vi "运维调试_CODMn.vi"() -> ()   [LabVIEW 2016, in "一代CodMn.lvlib"]
uses:
  <vilib>/Utility/miscctls.llb/LVPointTypeDef.ctl
panel:
  out "W7.13 加热超时":bool
  out "版本号":u32
  in  "滴定曲线界面返回":bool
  in  "滴定曲线":bool
  out "ORP滴定曲线":u16[](graph)
  out "滴定值":sgl
  out "硫酸计数":u16
  out "草酸钠计数":u16
  out "高锰酸钾计数":u16
  out "进样计数":u16
  out "运行步骤":u16(ring) items=["待机", "润洗", "进水样\\高锰酸钾\\加热", "进草酸钠", "高锰酸钾滴定", "排液"]
  out "运行计时分":u16 format="%02d"
  out "运行计时秒":u16 format="%02d"
  in  "标液浓度设置":sgl
  in  "零点滴定值设置":sgl
  in  "零点泵计量值设置":sgl
  in  "标度滴定值设置":sgl
  in  "标度泵计量值设置":sgl
  out "泵滴定数":sgl
  out "ORPK":sgl
  out "ORPB":sgl
  out "ORPA":sgl
  out "W7.12 校标错误":bool
  out "W7.11 校零错误":bool
  out "W7.10 测量错误":bool
  out "W7.07 草酸钠报警":bool
  out "W7.06 高锰酸钾报警":bool
  out "W7.02 加热超温":bool
  out "W7.01 温控器故障":bool
  out "W7.00 ORP故障":bool
  in  "清除报警":bool
  out "TempC":sgl
  out "ORP":i16
  in  "返回":bool
  in  "设置":bool
  out "运行状态":bool
  out "通讯状态":bool
  out "标样核查标记":bool
  out "空白核查标记":bool
  in  "标样核查":bool
  in  "空白核查":bool
  out "正在测量标记":bool
  out "CODMn浓度":sgl format="%.2f"
  out "校零标记":bool
  out "校标标记":bool
  out "故障标记":bool
  out "零点滴定值":sgl
  out "零点泵计量值":sgl
  out "标度滴定值":sgl
  out "标度泵计量值":sgl
  out "排液标记":bool
  in  "停止":bool
  in  "校准标度":bool
  in  "校准零点":bool
  in  "手动启动":bool
  # ":"
  # "运行计时:"
  # "CODMn"
  # "零点滴定值:"
  # "零点泵计量值:"
  # "标度滴定值:"
  # "标度泵计量值:"
  # "ORPA:"
  # "ORPB:"
  # "ORPK:"
  # "泵滴定数:"
  # "滴定值:"
  # "mg/L"
  # "标液浓度:"
  # "零点滴定值:"
  # "零点泵计量值:"
  # "标度滴定值:"
  # "标度泵计量值:"
  # "硫酸计数"
  # "草酸钠计数"
  # "高锰酸钾计数"
  # "进样计数"
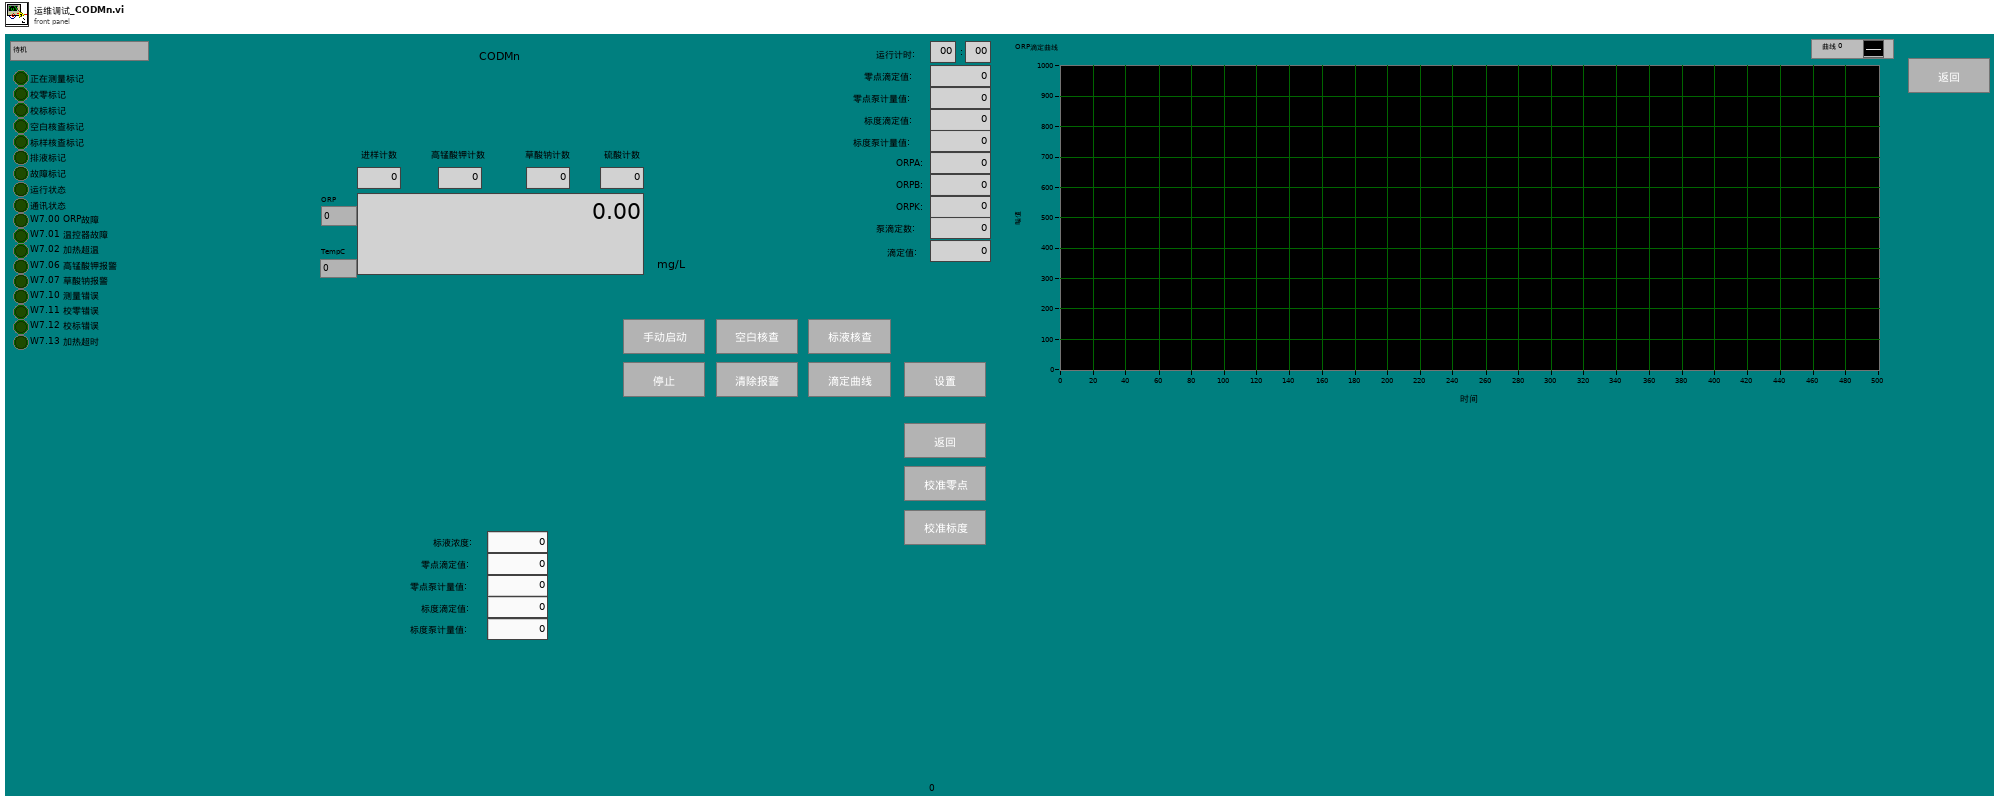
[diagram p1: front panel]
types:
  T1 = enum16{"open", "close", "readHR", "writeHR", "readCoil", "writeCoil"}
  T2 = typedef "LVPointTypeDef.ctl" = cluster{"Horizontal":i16, "Vertical":i16}
  T3 = enum16{"零点泵计量值设置", "零点滴定值设置", "标度泵计量值设置", "标度滴定值设定", "标液浓度设置"}
  T4 = enum16{"测量", "校零", "校标", "填充管路", "外部停止", "连续测量", "空白测量", "标样测量", "故障状态清除"}
  T5 = cluster{"时间标识":timestamp, "设备":string, "日志信息":string}
  T6 = cluster{"时间标识":timestamp, "设备":string, "日志信息":string, "流程参数":string}
  T7 = cluster{"时间":timestamp, "测量模式":string, "数据类型":string, "检测值":sgl, "单位":string, "数据标识":string, "因子编码":string, "标样参考值":sgl, "ORP-A":sgl, "ORP-B":sgl, "ORP-K":sgl, "COD滴定值":sgl, "高锰酸钾滴定数":sgl, "温度":sgl}
  T8 = enum8{"Enabled", "Disabled", "Disabled and Grayed Out"}
  T9 = cluster{"报警信息":cluster{"ORP故障":bool, "温控器故障":bool, "加热超温":bool, "水样报警":bool, "蒸馏水报警":bool, "标液报警":bool, "高锰酸钾报警":bool, "草酸钠报警":bool, "硫酸报警":bool, "硝酸银报警":bool, "测量错误":bool, "校零错误":bool, "校标错误":bool, "加热超时":bool, "待定2":bool, "待定3":bool}, "工作状态":cluster{"正在测量":bool, "校零标志":bool, "校标标志":bool, "排空标志":bool, "自动标志":bool, "增强校零":bool, "增强校标":bool, "停止标志":bool, "排废液":bool, "连续标志":bool, "量程50":bool, "量程100":bool, "自动计量调整":bool, "空白核查":bool, "标样核查":bool, "故障标志":bool}, "测量浓度值":sgl, "当前步序":u16, "当前ORP值":i16, "当前温度值":sgl, "零点滴定值":sgl, "零点泵计量值":i16, "标度滴定值":sgl, "标度泵计量值":i16, "ORPA":i16, "ORPB":i16, "ORPK":i16, "COD滴定值":sgl, "COD泵滴定数":u16, "标液浓度":sgl, "运行计时分":u16, "运行计时秒":u16, "进样计数":u16, "高锰酸钾计数":u16, "草酸钠计数":u16, "硫酸计数":u16, "版本号":u32}
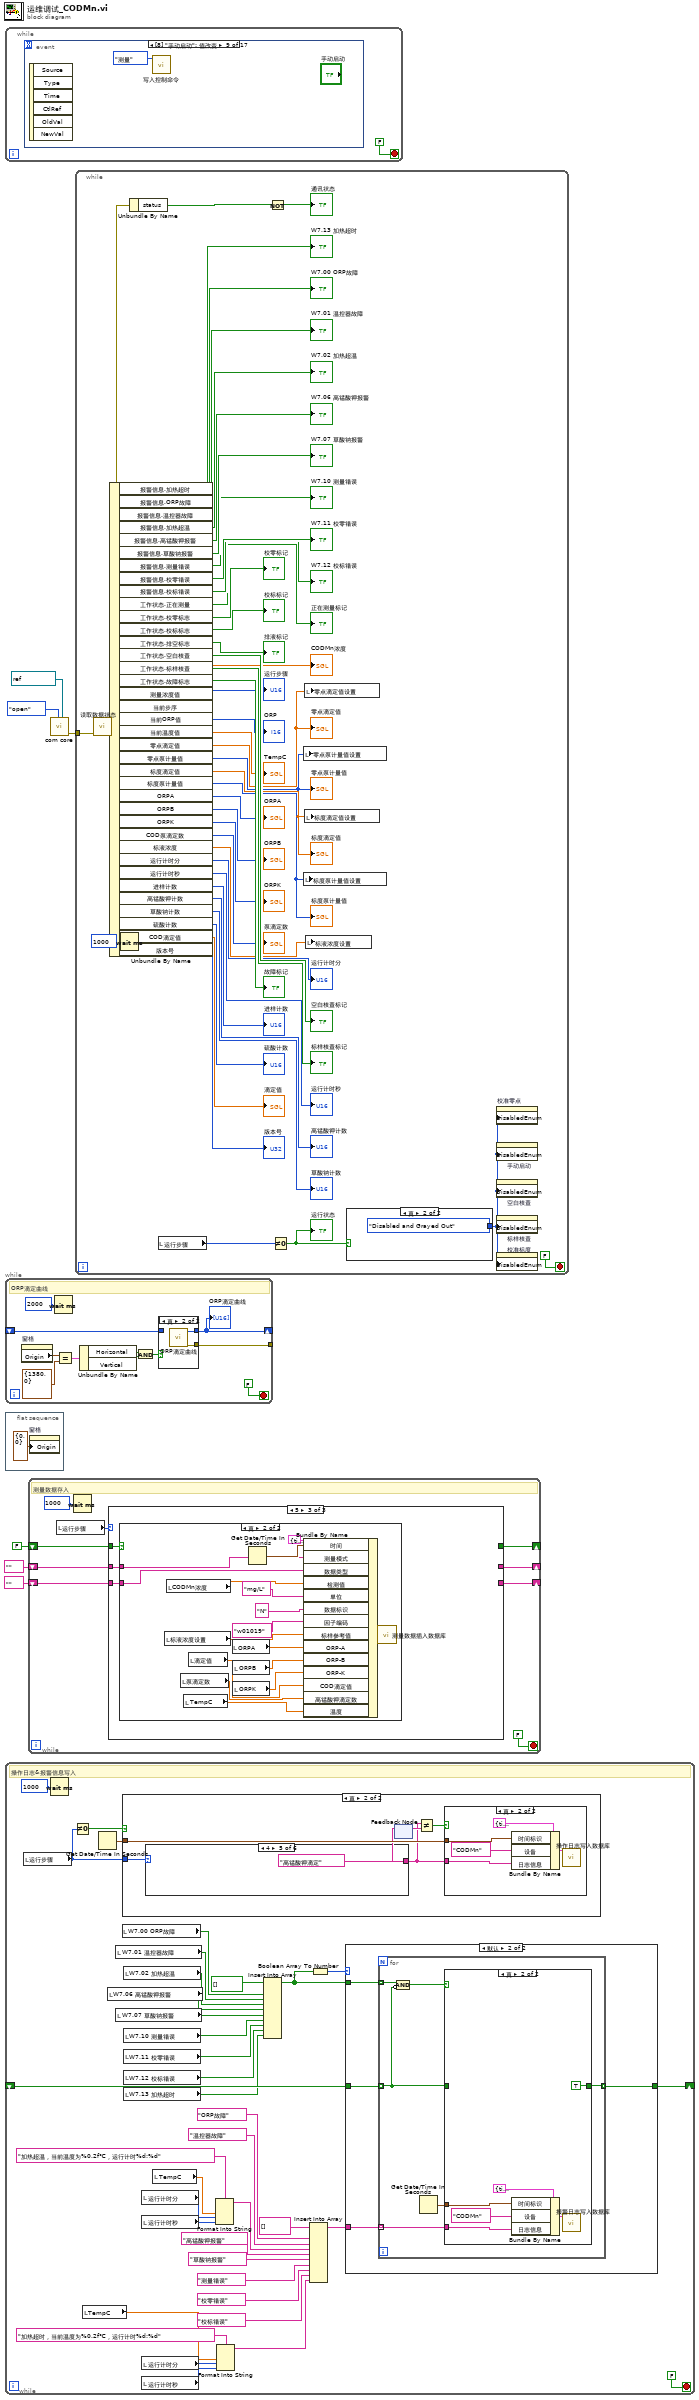
[diagram p0: block diagram]
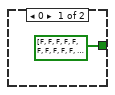
[diagram p3: hidden frame]
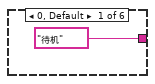
[diagram p7: hidden frame]
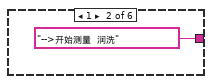
[diagram p8: hidden frame]
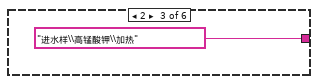
[diagram p9: hidden frame]
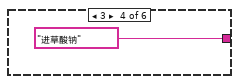
[diagram p10: hidden frame]
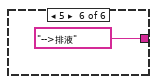
[diagram p11: hidden frame]
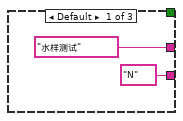
[diagram p12: hidden frame]
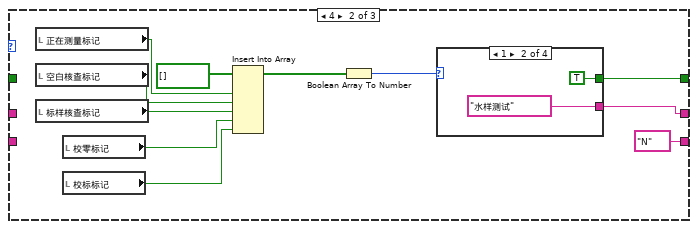
[diagram p13: hidden frame]
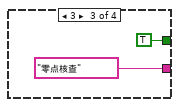
[diagram p15: hidden frame]
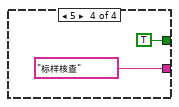
[diagram p16: hidden frame]
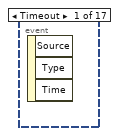
[diagram p19: hidden frame]
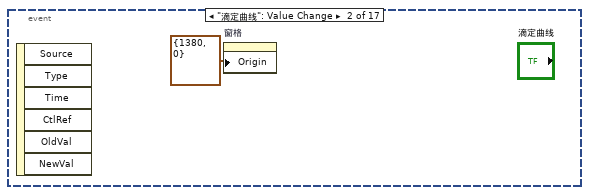
[diagram p20: hidden frame]
diagram:
  n1 = while {
    stop <- FALSE stop-if-true
    n2 = event shown="[8] \"手动启动\": 值改变" {
      selector: _ -> [_ _ _ _ _ _ _ _ _ _ _ _ _ _ _ _ _]
      dyn-events: _ -> [_ _ _ _ _ _ _ _ _ _ _ _ _ _ _ _ _]
      timeout: _ -> [_ _ _ _ _ _ _ _ _ _ _ _ _ _ _ _ _]
      event Timeout {
        n3 = event-data() -> ()  [unwired: 1 in, 3 out]
      }
      event "滴定曲线": Value Change {
        n4 = event-data() -> ()  [unwired: 1 in, 6 out]
        n5 = property on="窗格" class="Pane"("Origin"=T2 {"Horizontal"=1380, "Vertical"=0} ("原点")) -> ()  [unwired: 2 in, 2 out]
      }
      event "标度泵计量值设置", "标度滴定值设置", "零点泵计量值设置", "零点滴定值设置", "标液浓度设置": Mouse Down {
        n6 = event-data() -> ("CtlRef"=w13:refnum<vi>)  [unwired: 1 in, 5 out]
        n7 = property class="DigNum (严格)"(reference=w13) -> (reference out=w12:refnum<vi>, "Value"=w11:sgl)  [unwired: 1 in, 1 out]
        n8 = call "数字键盘.vi"("OldNumber"=w11) -> ("NewNumber"=w10:sgl)
        n9 = Not Equal?(x=w10, y=w11) -> (x != y?=w9:bool)
        n10 = case shown="真" w9 {
          tunnel: w12 -> [_ w15]
          tunnel: w10 -> [_ w14]
          frame False {
          }
          frame True {
            n11 = property class="DigNum (严格)"(reference=w15, "Val(Sgnl)"=w14) -> ()  [unwired: 1 in, 2 out]
          }
        }
      }
      event "标度泵计量值设置": Value Change {
        n12 = event-data() -> ()  [unwired: 1 in, 6 out]
        n13 = call "写入参数.vi"("写入参数"=T3."标度泵计量值设置", "写入值"="标度泵计量值设置") -> ()  [unwired: 9 in, 1 out]
      }
      event "标度滴定值设置": Value Change {
        n14 = event-data() -> ()  [unwired: 1 in, 6 out]
        n15 = call "写入参数.vi"("写入参数"=T3."标度滴定值设定", "写入值"="标度滴定值设置") -> ()  [unwired: 9 in, 1 out]
      }
      event "零点泵计量值设置": Value Change {
        n16 = event-data() -> ()  [unwired: 1 in, 6 out]
        n17 = call "写入参数.vi"("写入参数"=T3."零点泵计量值设置", "写入值"="零点泵计量值设置") -> ()  [unwired: 9 in, 1 out]
      }
      event "零点滴定值设置": Value Change {
        n18 = event-data() -> ()  [unwired: 1 in, 6 out]
        n19 = call "写入参数.vi"("写入参数"=T3."零点滴定值设置", "写入值"="零点滴定值设置") -> ()  [unwired: 9 in, 1 out]
      }
      event "标液浓度设置": Value Change {
        n20 = event-data() -> ()  [unwired: 1 in, 6 out]
        n21 = call "写入参数.vi"("写入参数"=T3."标液浓度设置", "写入值"="标液浓度设置") -> ()  [unwired: 9 in, 1 out]
      }
      event "手动启动": Value Change {
        n22 = event-data() -> ()  [unwired: 1 in, 6 out]
        n23 = call "写入控制命令.vi"("命令"=T4."测量") -> ()  [unwired: 10 in, 1 out]
      }
      event "空白核查": Value Change {
        n24 = event-data() -> ()  [unwired: 1 in, 6 out]
        n25 = call "写入控制命令.vi"("命令"=T4."空白测量") -> ()  [unwired: 10 in, 1 out]
      }
      event "标样核查": Value Change {
        n26 = event-data() -> ()  [unwired: 1 in, 6 out]
        n27 = call "写入控制命令.vi"("命令"=T4."标样测量") -> ()  [unwired: 10 in, 1 out]
      }
      event "设置": Value Change {
        n28 = event-data() -> ()  [unwired: 1 in, 6 out]
        n29 = property on="窗格" class="Pane"("Origin"=T2 {"Horizontal"=0, "Vertical"=528} ("原点")) -> ()  [unwired: 2 in, 2 out]
      }
      event "返回", "滴定曲线界面返回": Value Change {
        n30 = event-data() -> ()  [unwired: 1 in, 6 out]
        n31 = property on="窗格" class="Pane"("Origin"=T2 {"Horizontal"=0, "Vertical"=0} ("原点")) -> ()  [unwired: 2 in, 2 out]
      }
      event "校准零点": Value Change {
        n32 = event-data() -> ()  [unwired: 1 in, 3 out]
        n33 = call "写入控制命令.vi"("命令"=T4."校零") -> ()  [unwired: 10 in, 1 out]
      }
      event "校准标度": Value Change {
        n34 = event-data() -> ()  [unwired: 1 in, 3 out]
        n35 = call "写入控制命令.vi"("命令"=T4."校标") -> ()  [unwired: 10 in, 1 out]
      }
      event "停止": Value Change {
        n36 = event-data() -> ()  [unwired: 1 in, 3 out]
        n37 = call "写入控制命令.vi"("命令"=T4."外部停止") -> ()  [unwired: 10 in, 1 out]
      }
      event "清除报警": Value Change {
        n38 = event-data() -> ()  [unwired: 1 in, 6 out]
        n39 = call "写入控制命令.vi"("命令"=T4."故障状态清除") -> ()  [unwired: 10 in, 1 out]
      }
    }
  }
  n40 = while {
    shift-right: [w40] -> _
    shift-left: _ -> [w41]
    tunnel: [w35] -> _
    stop <- FALSE stop-if-true
    # "ORP滴定曲线"
    n41 = property on="窗格" class="Pane"() -> ("Origin"=w44:T2)  [unwired: 2 in, 2 out]
    n42 = Wait (ms)(milliseconds to wait=u32 2000 ("等待时间（毫秒）")) -> ()  [unwired: 1 out]
    n43 = Equal?(x=w44, y=T2 {"Horizontal"=1380, "Vertical"=0}) -> (x = y?=w42:cluster{"Horizontal":bool, "Vertical":bool})
    n44 = Unbundle By Name(w42) -> ("Horizontal"=w37:bool, "Vertical"=w38:bool)
    n45 = And(x=w37, y=w38) -> (x .and. y?=w36:bool)
    n46 = case shown="真" w36 {
      tunnel: [w46 w48] -> w40
      tunnel: w41 -> [w46 _]
      tunnel: [_ w47] -> w35
      frame False {
      }
      frame True {
        n47 = call "ORP滴定曲线.vi"() -> ("error out"=w47:errorcluster, "输出数组"=w48:u16[])  [unwired: 10 in]
      }
    }
    "ORP滴定曲线" <- w40
  }
  n48 = flat-sequence {
    frame #0 {
      n49 = property on="窗格" class="Pane"("Origin"=T2 {"Horizontal"=0, "Vertical"=0} ("原点")) -> ()  [unwired: 2 in, 2 out]
    }
  }
  n50 = while {
    shift-right: [w62] -> _
    shift-left: _ -> [w61]
    stop <- FALSE stop-if-true
    # "操作日志&报警信息写入"
    n51 = local read "运行步骤"() -> (w84:u16)
    n52 = Wait (ms)(milliseconds to wait=u32 1000 ("等待时间（毫秒）")) -> ()  [unwired: 1 out]
    n53 = Not Equal To 0?(x=w84) -> (x != 0?=w85:bool)
    n54 = local read "TempC"() -> (w50:sgl)
    n55 = Get Date/Time In Seconds() -> (seconds since 1Jan1904=w83:timestamp)
    n56 = local read "W7.06 高锰酸钾报警"() -> (w79:bool)
    n57 = local read "W7.01 温控器故障"() -> (w81:bool)
    n58 = local read "W7.07 草酸钠报警"() -> (w78:bool)
    n59 = local read "W7.00 ORP故障"() -> (w82:bool)
    n60 = case shown="真" w85 {
      tunnel: w84 -> [_ w110]
      tunnel: w83 -> [_ w109]
      frame False {
      }
      frame True {
        n61 = case shown="4" w110 {
          tunnel: ["待机" ("操作步骤") "-->开始测量  润洗" ("操作步骤") "进水样\\高锰酸钾\\加热" ("操作步骤") "进草酸钠" ("操作步骤") "高锰酸钾滴定" ("操作步骤") "-->排液" ("操作步骤")] -> w106
          frame 0, Default {
          }
          frame 1 {
          }
          frame 2 {
          }
          frame 3 {
          }
          frame 4 {
          }
          frame 5 {
          }
        }
        n62 = feedback-in #1(w106) -> ()
        n63 = feedback #1() -> (w108:string)  [unwired: 1 in]
        n64 = Not Equal?(x=w106, y=w108) -> (x != y?=w107:bool)
        n65 = case shown="真" w107 {
          tunnel: w109 -> [_ w115]
          tunnel: w106 -> [_ w114]
          frame False {
          }
          frame True {
            n66 = Bundle By Name(cluster=T6 {"时间标识"=timestamp(0 s since 1904-01-01), "设备"="", "日志信息"="", "流程参数"=""} ("data in"), "时间标识"=w115, "设备"="CODMn", "日志信息"=w114) -> (w111:T6)
            n67 = call "操作日志写入数据库.vi"("data in"=w111) -> ()  [unwired: 10 in, 1 out]
          }
        }
      }
    }
    n68 = local read "W7.02 加热超温"() -> (w80:bool)
    n69 = local read "W7.10 测量错误"() -> (w77:bool)
    n70 = local read "W7.11 校零错误"() -> (w76:bool)
    n71 = local read "W7.12 校标错误"() -> (w75:bool)
    n72 = local read "W7.13 加热超时"() -> (w60:bool)
    n73 = local read "运行计时分"() -> (w56:u16)
    n74 = local read "运行计时秒"() -> (w55:u16)
    n75 = local read "运行计时分"() -> (w53:u16)
    n76 = local read "运行计时秒"() -> (w54:u16)
    n77 = local read "TempC"() -> (w59:sgl)
    n78 = Format Into String(format string="加热超温，当前温度为%0.2f℃，运行计时%d:%d" ("格式字符串"), w59, w56, w55) -> (resulting string=w57:string)  [unwired: 2 in, 1 out]
    n79 = Format Into String(format string="加热超时，当前温度为%0.2f℃，运行计时%d:%d" ("格式字符串"), w50, w53, w54) -> (resulting string=w51:string)  [unwired: 2 in, 1 out]
    n80 = Insert Into Array(array=bool[] [] ("数组"), new element #1=w82, new element #2=w81, new element #3=w80, new element #4=w79, new element #5=w78, new element #6=w77, new element #7=w76, new element #8=w75, new element #9=w60) -> (w64:bool[])  [unwired: 1 in]
    n81 = Insert Into Array(array=string[] [] ("数组"), new element #1="ORP故障" ("组合框"), new element #2="温控器故障" ("组合框"), new element #3=w57, new element #4="高锰酸钾报警" ("组合框"), new element #5="草酸钠报警" ("组合框"), new element #6="测量错误" ("组合框"), new element #7="校零错误" ("组合框"), new element #8="校标错误" ("组合框"), new element #9=w51) -> (w65:string[])  [unwired: 1 in]
    n82 = Boolean Array To Number(Boolean array=w64) -> (number=w63:u32)
    n83 = case shown="默认" w63 {
      tunnel: w65 -> [_ w92]
      tunnel: w64 -> [_ w91]
      tunnel: [bool[] [FALSE, FALSE, FALSE, FALSE, FALSE, FALSE, FALSE, FALSE, FALSE, FALSE, FALSE, FALSE, FALSE, FALSE, FALSE, FALSE] w90] -> w62
      tunnel: w61 -> [_ w89]
      frame 0 {
      }
      frame Default {
        n84 = for {
          tunnel: w91 -> [w95] mode=indexing
          tunnel: w92 -> [w97] mode=indexing
          tunnel: [w96] -> w90 mode=indexing
          tunnel: w89 -> [w93] mode=indexing
          n85 = Compound Arithmetic op=AND ("复合运算")(w95, invert w93) -> (w94:bool)
          n86 = Get Date/Time In Seconds() -> (seconds since 1Jan1904=w98:timestamp)
          n87 = case shown="真" w94 {
            tunnel: w98 -> [_ w103]
            tunnel: w97 -> [_ w101]
            tunnel: [w99 TRUE ("W7.12 校标错误")] -> w96
            tunnel: w93 -> [w99 _]
            frame False {
            }
            frame True {
              n88 = Bundle By Name(cluster=T5 {"时间标识"=timestamp(0 s since 1904-01-01), "设备"="", "日志信息"=""} ("data in"), "时间标识"=w103, "设备"="CODMn", "日志信息"=w101) -> (w104:T5)
              n89 = call "报警日志写入数据库.vi"("data in"=w104) -> ()  [unwired: 10 in, 1 out]
            }
          }
        }
      }
    }
  }
  n90 = while {
    shift-right: [w127] -> _
    shift-left: FALSE -> [w128]
    shift-right: [w123] -> _
    shift-left: "" ("测量模式") -> [w125]
    shift-right: [w122] -> _
    shift-left: "" ("数据类型") -> [w124]
    stop <- FALSE stop-if-true
    # "测量数据存入"
    n91 = local read "运行步骤"() -> (w129:u16)
    n92 = Wait (ms)(milliseconds to wait=u32 1000 ("等待时间（毫秒）")) -> ()  [unwired: 1 out]
    n93 = case shown="5" w129 {
      tunnel: w128 -> [_ _ w152]
      tunnel: [_ w133 _] -> w127
      tunnel: w125 -> [_ _ w151]
      tunnel: w124 -> [_ _ w150]
      tunnel: ["水样测试" ("测量模式") w134 _] -> w123
      tunnel: ["N" ("数据类型") "N" ("数据类型") _] -> w122
      frame Default {
      }
      frame 4 {
        n94 = local read "正在测量标记"() -> (w142:bool)
        n95 = local read "空白核查标记"() -> (w140:bool)
        n96 = local read "标样核查标记"() -> (w139:bool)
        n97 = local read "校零标记"() -> (w136:bool)
        n98 = local read "校标标记"() -> (w135:bool)
        n99 = Insert Into Array(array=bool[] [] ("数组"), new element #1=w142, new element #2=w140, new element #3=w139, new element #4=w136, new element #5=w135) -> (w138:bool[])  [unwired: 1 in]
        n100 = Boolean Array To Number(Boolean array=w138) -> (number=w137:u32)
        n101 = case shown="1" w137 {
          tunnel: [_ "水样测试" ("测量模式") "零点核查" ("测量模式") "标样核查" ("测量模式")] -> w134
          tunnel: [_ TRUE TRUE TRUE] -> w133
          frame 0, Default {
          }
          frame 1 {
          }
          frame 3 {
          }
          frame 5 {
          }
        }
      }
      frame 5 {
        n102 = case shown="真" w152 {
          tunnel: w151 -> [_ w162]
          tunnel: w150 -> [_ w161]
          frame False {
          }
          frame True {
            n103 = local read "标液浓度设置"() -> (w159:sgl)
            n104 = local read "CODMn浓度"() -> (w160:sgl)
            n105 = local read "泵滴定数"() -> (w154:sgl)
            n106 = local read "TempC"() -> (w153:sgl)
            n107 = local read "滴定值"() -> (w155:sgl)
            n108 = local read "ORPA"() -> (w158:sgl)
            n109 = local read "ORPB"() -> (w157:sgl)
            n110 = local read "ORPK"() -> (w156:sgl)
            n111 = Get Date/Time In Seconds() -> (seconds since 1Jan1904=w166:timestamp)
            n112 = Bundle By Name(cluster=T7 {"时间"=timestamp(0 s since 1904-01-01), "测量模式"="", "数据类型"="", "检测值"=0.0, "单位"="mg/L", "数据标识"="N", "因子编码"="w01019", "标样参考值"=0.0, "ORP-A"=0.0, "ORP-B"=0.0, "ORP-K"=0.0, "COD滴定值"=0.0, "高锰酸钾滴定数"=0.0, "温度"=0.0} ("data"), "时间"=w166, "测量模式"=w162, "数据类型"=w161, "检测值"=w160, "单位"="mg/L", "数据标识"="N", "因子编码"="w01019", "标样参考值"=w159, "ORP-A"=w158, "ORP-B"=w157, "ORP-K"=w156, "COD滴定值"=w155, "高锰酸钾滴定数"=w154, "温度"=w153) -> (w167:T7)
            n113 = call "测量数据插入数据库.vi"("data"=w167) -> ()  [unwired: 10 in, 1 out]
          }
        }
      }
    }
  }
  n114 = call "com core.vi"("VISA Resource"=refnum<visa-resource-name> "COM3", "功能"=T1."open") -> ("error out"=w5:errorcluster)  [unwired: 7 in, 2 out]
  n115 = while {
    tunnel: w5 -> [w212]
    stop <- FALSE stop-if-true
    n116 = call "读取数据状态.vi"("error in (no error)"=w212) -> ("error out"=w202:errorcluster, "簇"=w211:T9)  [unwired: 9 in]
    n117 = Unbundle By Name(w211) -> ("报警信息.加热超时"=→"W7.13 加热超时":bool, "报警信息.ORP故障"=→"W7.00 ORP故障":bool, "报警信息.温控器故障"=→"W7.01 温控器故障":bool, "报警信息.加热超温"=→"W7.02 加热超温":bool, "报警信息.高锰酸钾报警"=→"W7.06 高锰酸钾报警":bool, "报警信息.草酸钠报警"=→"W7.07 草酸钠报警":bool, "报警信息.测量错误"=→"W7.10 测量错误":bool, "报警信息.校零错误"=→"W7.11 校零错误":bool, "报警信息.校标错误"=→"W7.12 校标错误":bool, "工作状态.正在测量"=→"正在测量标记":bool, "工作状态.校零标志"=→"校零标记":bool, "工作状态.校标标志"=→"校标标记":bool, "工作状态.排空标志"=→"排液标记":bool, "工作状态.空白核查"=→"空白核查标记":bool, "工作状态.标样核查"=→"标样核查标记":bool, "工作状态.故障标志"=→"故障标记":bool, "测量浓度值"=→"CODMn浓度":sgl, "当前步序"=→"运行步骤":u16, "当前ORP值"=→"ORP":i16, "当前温度值"=→"TempC":sgl, "零点滴定值"=w183:sgl, "零点泵计量值"=w182:i16, "标度滴定值"=w181:sgl, "标度泵计量值"=w180:i16, "ORPA"=→"ORPA":i16, "ORPB"=→"ORPB":i16, "ORPK"=→"ORPK":i16, "COD泵滴定数"=→"泵滴定数":u16, "标液浓度"=w184:sgl, "运行计时分"=→"运行计时分":u16, "运行计时秒"=→"运行计时秒":u16, "进样计数"=→"进样计数":u16, "高锰酸钾计数"=→"高锰酸钾计数":u16, "草酸钠计数"=→"草酸钠计数":u16, "硫酸计数"=→"硫酸计数":u16, "COD滴定值"=→"滴定值":sgl, "版本号"=→"版本号":u32)
    "零点滴定值" <- w183
    "零点泵计量值" <- w182
    "标度滴定值" <- w181
    "标度泵计量值" <- w180
    n118 = Wait (ms)(milliseconds to wait=u32 1000 ("等待时间（毫秒）")) -> ()  [unwired: 1 out]
    n119 = Unbundle By Name(w202) -> ("status"=w201:bool)
    n120 = local read "运行步骤"() -> (w176:u16)
    n121 = Not(x=w201) -> (.not. x?=→"通讯状态":bool)
    n122 = Not Equal To 0?(x=w176) -> (x != 0?=w185:bool)
    "运行状态" <- w185
    n123 = local write "零点泵计量值设置"(w182) -> ()
    n124 = local write "标度泵计量值设置"(w180) -> ()
    n125 = local write "零点滴定值设置"(w183) -> ()
    n126 = local write "标度滴定值设置"(w181) -> ()
    n127 = local write "标液浓度设置"(w184) -> ()
    n128 = case shown="真" w185 {
      tunnel: [_ T8."Disabled and Grayed Out" ("禁用")] -> w213
      frame False {
      }
      frame True {
      }
    }
    n129 = property on="校准零点" class="Bool"("DisabledEnum"=w213) -> ()  [unwired: 2 in, 2 out]
    n130 = property on="手动启动" class="Bool"("DisabledEnum"=w213) -> ()  [unwired: 2 in, 2 out]
    n131 = property on="空白核查" class="Bool"("DisabledEnum"=w213) -> ()  [unwired: 2 in, 2 out]
    n132 = property on="标样核查" class="Bool"("DisabledEnum"=w213) -> ()  [unwired: 2 in, 2 out]
    n133 = property on="校准标度" class="Bool"("DisabledEnum"=w213) -> ()  [unwired: 2 in, 2 out]
  }
